vi "Show test result.vi"(8 "error in (no error)":errorcluster) -> (0 "error out":errorcluster)   [LabVIEW 2013]
uses:
  <vilib>/event_ctls.llb/eventvkey.ctl
  Main Support/Global 2.vi
  Test Globals/Global 1.vi
panel:
  out "Message":string
  # "Test Result Message"
  # "Press SPACE BAR to continue"
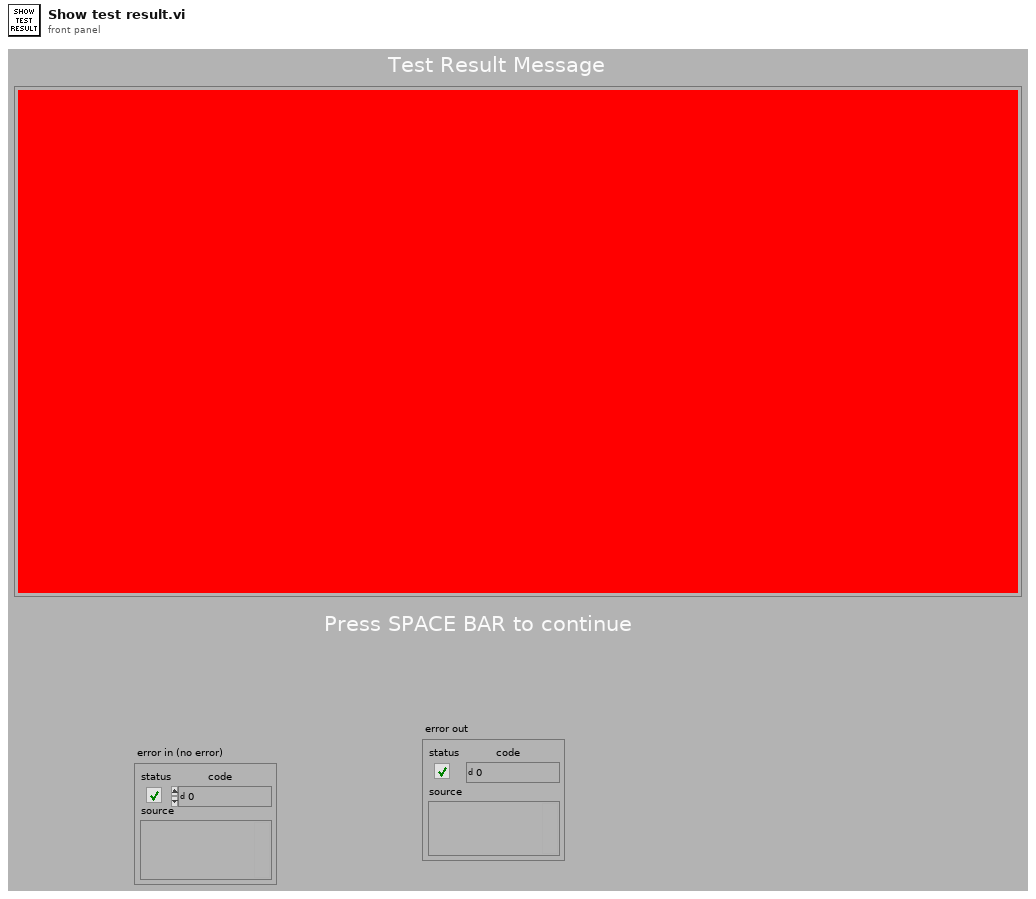
[diagram p1: front panel]
types:
  T1 = typedef "eventvkey.ctl" = enum16{"ASCII", "Enter", "Return", "Shift", "Ctrl", "Alt", "Cmd", "Opt", "Caps", "NumLock", "Clear", "Break", "Up", "Down", "Left", "Right", "Insert", "Delete", "Home", "End", "PageUp", "PageDown", "Escape", "Help", "Pause", "ScrollLock", "F1", "F2", "F3", "F4", "F5", "F6", "F7", "F8", "F9", "F10", "F11", "F12", "F13", "F14", "F15", "F16", "F17", "F18", "F19", "F20", "F21", "F22", "F23", "F24", "Play", "VolumeUp", "VolumeDown", "Mute", "Two Byte Char"}
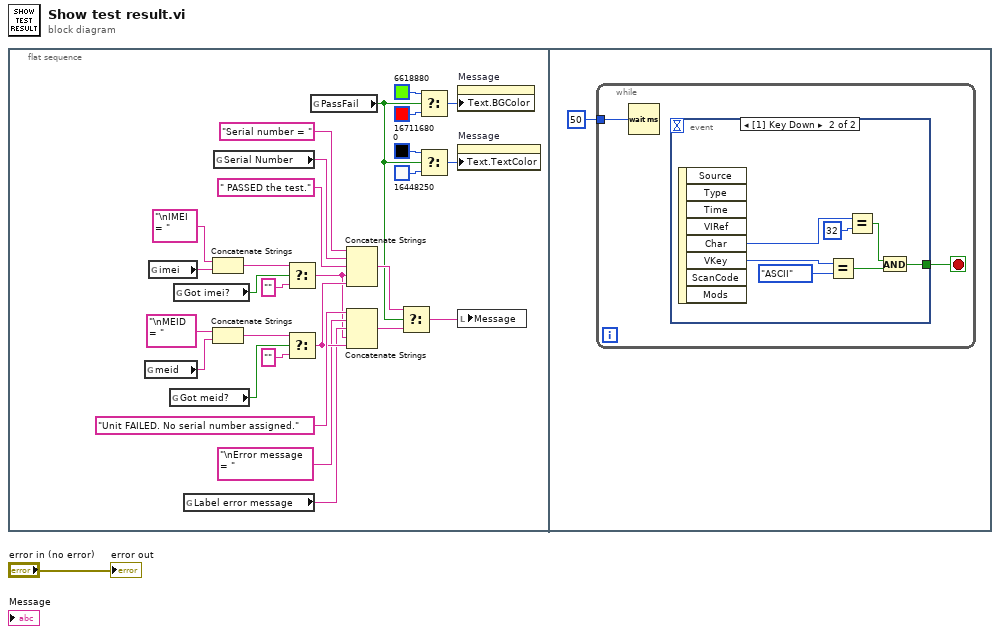
[diagram p0: block diagram]
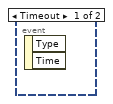
[diagram p2: hidden frame]
diagram:
  n1 = flat-sequence {
    frame #0 {
      n2 = global read "Global 1.vi" "meid"() -> (w10:string)
      n3 = global read "Global 1.vi" "imei"() -> (w14:string)
      n4 = global read "Global 1.vi" "Got meid?"() -> (w17:bool)
      n5 = global read "Global 1.vi" "Got imei?"() -> (w16:bool)
      n6 = global read "Global 1.vi" "Label error message"() -> (w3:string)
      n7 = Concatenate Strings("\nIMEI = ", w14) -> (w13:string)
      n8 = Concatenate Strings("\nMEID = ", w10) -> (w9:string)
      n9 = global read "Global 2.vi" "Serial Number"() -> (w28:string)
      n10 = Select(t=w13, s=w16, f="" ("y")) -> (s? t:f=w2:string)
      n11 = Select(t=w9, s=w17, f="" ("y")) -> (s? t:f=w6:string)
      n12 = global read "Global 2.vi" "PassFail"() -> (w20:bool)
      n13 = Concatenate Strings("Serial number = " ("string"), w28, " PASSED the test." ("string"), w2, w6) -> (w26:string)
      n14 = Concatenate Strings("Unit FAILED. No serial number assigned." ("f"), "\nError message = " ("string"), w3, w2, w6) -> (w5:string)
      n15 = Select(t=w26, s=w20, f=w5) -> (s? t:f=w25:string)
      n16 = Select(t=u32 6618880, s=w20, f=u32 16711680) -> (s? t:f=w18:u32)
      n17 = Select(t=u32 0, s=w20, f=u32 16448250) -> (s? t:f=w19:u32)
      n18 = property on="Message" class="Str"("Text.BGColor"=w18) -> ()  [unwired: 2 in, 2 out]
      n19 = property on="Message" class="Str"("Text.TextColor"=w19) -> ()  [unwired: 2 in, 2 out]
      n20 = local write "Message"(w25) -> ()
    }
    frame #1 {
      n21 = while {
        tunnel: u32 50 ("milliseconds to wait") -> [w32]
        stop <- w31 stop-if-true
        n22 = Wait (ms)(milliseconds to wait=w32) -> ()  [unwired: 1 out]
        n23 = event shown="[1] Key Down" {
          selector: _ -> [_ _]
          dyn-events: _ -> [_ _]
          timeout: _ -> [_ _]
          tunnel: [_ w33] -> w31
          event Timeout {
            n24 = event-data() -> ()  [unwired: 1 in, 2 out]
          }
          event Key Down {
            n25 = event-data() -> ("Char"=w39:i16, "VKey"=w37:T1)  [unwired: 1 in, 6 out]
            n26 = Equal?(x=w37, y=eventvkey."ASCII" ("VKey")) -> (x = y?=w34:bool)
            n27 = Equal?(x=w39, y=i16 32) -> (x = y?=w35:bool)
            n28 = And(x=w35, y=w34) -> (x .and. y?=w33:bool)
          }
        }
      }
    }
  }
  "error out" <- "error in (no error)"
